vi "Auto Near Switch.vi"(10 "Right?":bool) -> ()   [LabVIEW 2017]
uses:
  Auto switch direita.ctl
  LabVIEW_is_Under_Control.lib/Util/Unpack Gamepad/Button Cluster.ctl
  Team Code/Robot Global Data.vi
panel:
  in  "Delay fwd 2":i32=200
  in  "DistanceAfterTurn":dbl=40.0
  in  "Delay Turn":i32=200
  in  "Turn":dbl=-90.0 format="%#_13g"
  in  "Time to wait (min 50ms)":dbl=50.0
  in  "Delay Fwd":i32=500
  in  "DistanceSwitch":dbl=400.0
  out "auto state":T1=enum."Girando"
  # "AINDA FALTA ADCIONAR:\n\n- Gatilho que troque de estado caso o tempo limite tenha passado\n\n-Algo que detecte um mal funcionamento do navx, e ignore o sinal dele para fazer o auto."
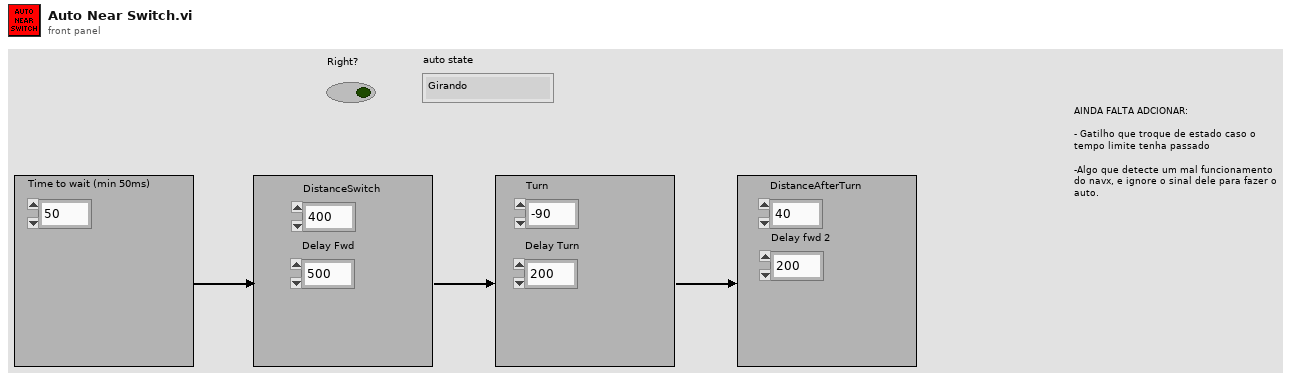
[diagram p1: front panel]
types:
  T1 = typedef "Auto switch direita.ctl" = enum16{"Zerandosensor", "Girando", "Andando", "Jogando", "Andando2", "Finalizando", "Zerandosensor2"}
  T2 = cluster{"proportional gain (Kc)":dbl, "integral time (Ti, min)":dbl, "derivative time (Td, min)":dbl}
  T3 = typedef "Button Cluster.ctl" = cluster{"Buttons[0]":bool, "Buttons[1]":bool, "Buttons[2]":bool, "Buttons[3]":bool, "Buttons[4]":bool, "Buttons[5]":bool, "Buttons[6]":bool, "Buttons[7]":bool, "Buttons[8]":bool, "Buttons[9]":bool}
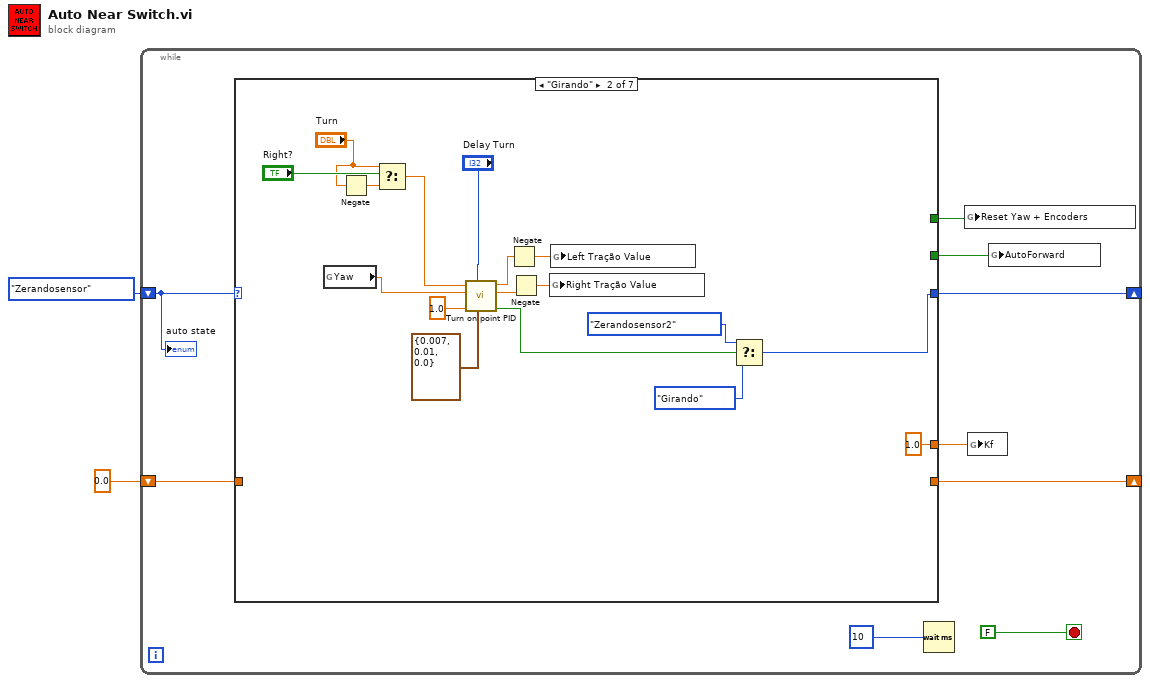
[diagram p0: block diagram]
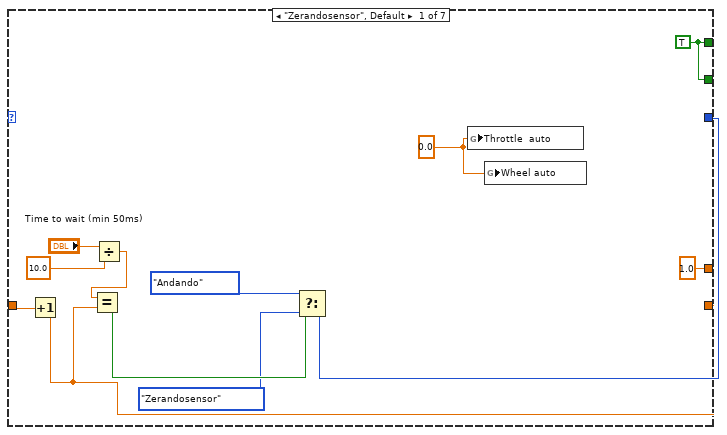
[diagram p2: hidden frame]
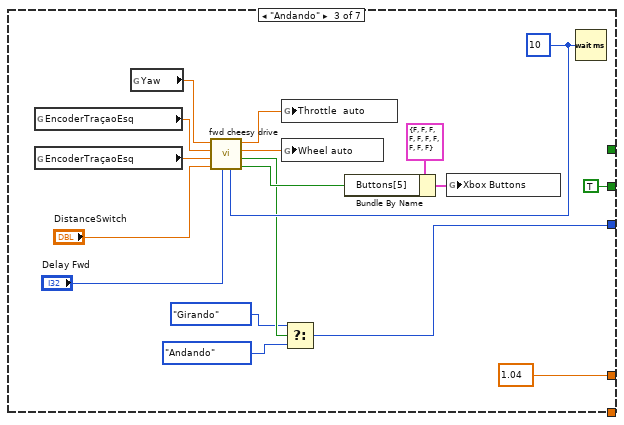
[diagram p3: hidden frame]
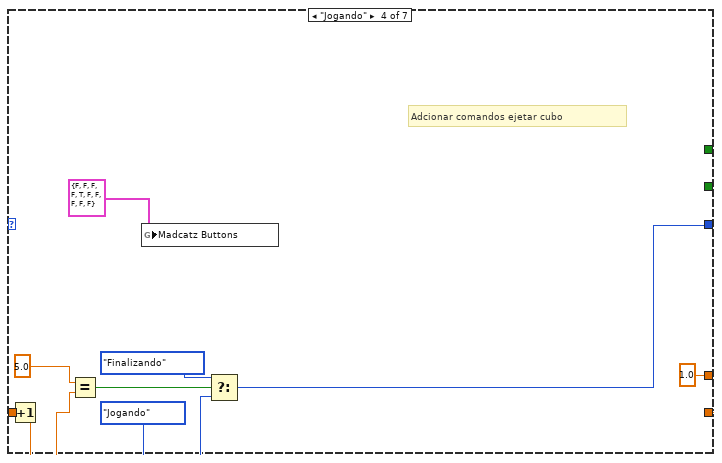
[diagram p4: hidden frame]
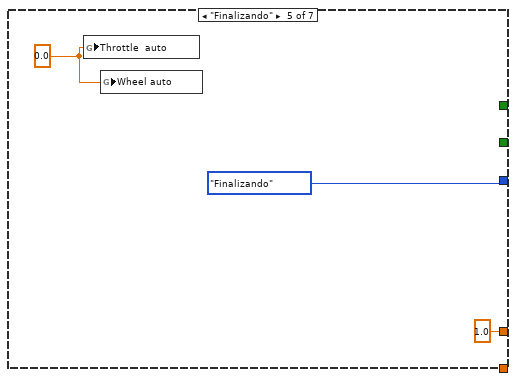
[diagram p5: hidden frame]
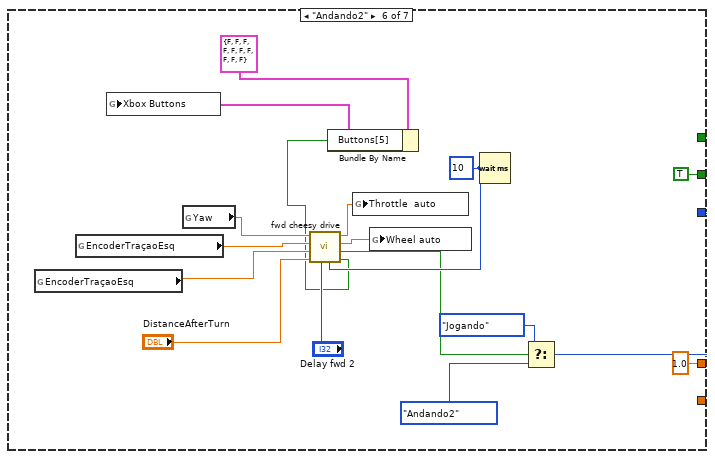
[diagram p6: hidden frame]
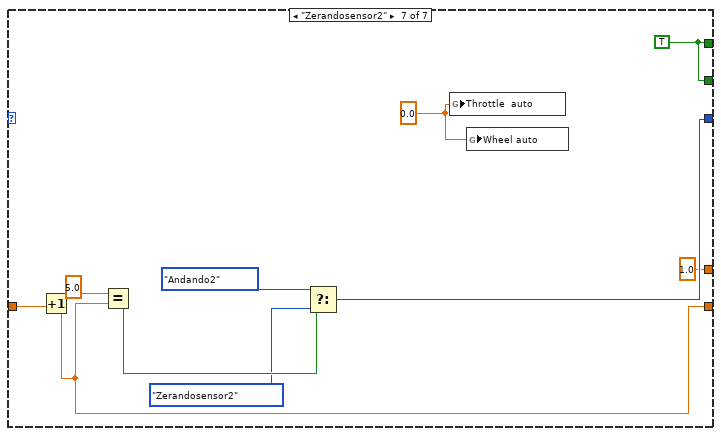
[diagram p7: hidden frame]
diagram:
  n1 = while {
    shift-right: [w7] -> _
    shift-left: Auto_switch_direita."Zerandosensor" -> [w5]
    shift-right: [w8] -> _
    shift-left: 0.0 -> [w9]
    stop <- FALSE stop-if-true
    n2 = case shown="\"Girando\"" w5 {
      tunnel: w9 -> [w23 _ _ w65 _ _ w88]
      tunnel: [w21 _ _ w62 _ _ w89] -> w8
      tunnel: [w20 w38 w45 w61 Auto_switch_direita."Finalizando" w72 w90] -> w7
      tunnel: [w17 _ _ _ _ _ w95] -> w4
      tunnel: [w17 _ TRUE _ _ TRUE w95] -> w6
      tunnel: [1.0 1.0 1.04 1.0 1.0 1.0 1.0] -> w3
      frame "Zerandosensor", Default {
        w16 = 0.0
        w17 = TRUE
        n3 = Increment(x=w23) -> (x+1=w21:dbl)
        n4 = Divide(x="Time to wait (min 50ms)", y=10.0) -> (x/y=w12:dbl)
        n5 = Equal?(x=w12, y=w21) -> (x = y?=w22:bool)
        n6 = Select(t=Auto_switch_direita."Andando", s=w22, f=Auto_switch_direita."Zerandosensor") -> (s? t:f=w20:T1)
        n7 = global write "Robot Global Data.vi" "Throttle  auto"(w16) -> ()
        n8 = global write "Robot Global Data.vi" "Wheel auto"(w16) -> ()
      }
      frame "Girando" {
        n9 = global read "Robot Global Data.vi" "Yaw"() -> (w31:dbl)
        n10 = Negate(x="Turn") -> (-x=w26:dbl)
        n11 = Select(t="Turn", s="Right?", f=w26) -> (s? t:f=w24:dbl)
        n12 = call "Turn on point PID.vi"("Gains"=T2 {"proportional gain (Kc)"=0.007, "integral time (Ti, min)"=0.01, "derivative time (Td, min)"=0.0}, "Time to stop"="Delay Turn", "Precision"=1.0, "Yaw"=w31, "Setpoint(degrees)"=w24) -> ("Finished?"=w39:bool, "PWM right"=w34:dbl, "PWM left"=w35:dbl)  [unwired: 4 in]
        n13 = Negate(x=w35) -> (-x=w30:dbl)
        n14 = Negate(x=w34) -> (-x=w29:dbl)
        n15 = global write "Robot Global Data.vi" "Right Tração Value"(w29) -> ()
        n16 = global write "Robot Global Data.vi" "Left Tração Value"(w30) -> ()
        n17 = Select(t=Auto_switch_direita."Zerandosensor2", s=w39, f=Auto_switch_direita."Girando") -> (s? t:f=w38:T1)
      }
      frame "Andando" {
        w53 = u32 10 ("milliseconds to wait")
        n18 = global read "Robot Global Data.vi" "EncoderTraçaoEsq"() -> (w55:dbl)
        n19 = global read "Robot Global Data.vi" "EncoderTraçaoEsq"() -> (w56:dbl)
        n20 = global read "Robot Global Data.vi" "Yaw"() -> (w57:dbl)
        n21 = call "fwd cheesy drive.vi"("Loop Timer"=w53, "Time to stop"="Delay Fwd", "Distance"="DistanceSwitch", "Encoder Left"=w56, "Encoder Right"=w55, "Yaw"=w57) -> ("Finished distance"=w47:bool, "Both finished"=w46:bool, "Direction"=w51:dbl, "Trottle"=w50:dbl)  [unwired: 2 in]
        n22 = global write "Robot Global Data.vi" "Throttle  auto"(w50) -> ()
        n23 = global write "Robot Global Data.vi" "Wheel auto"(w51) -> ()
        n24 = Select(t=Auto_switch_direita."Girando", s=w46, f=Auto_switch_direita."Andando") -> (s? t:f=w45:T1)
        n25 = Bundle By Name(cluster=T3 {"Buttons[0]"=FALSE, "Buttons[1]"=FALSE, "Buttons[2]"=FALSE, "Buttons[3]"=FALSE, "Buttons[4]"=FALSE, "Buttons[5]"=FALSE, "Buttons[6]"=FALSE, "Buttons[7]"=FALSE, "Buttons[8]"=FALSE, "Buttons[9]"=FALSE} ("Xbox Buttons"), "Buttons[5]"=w47) -> (w48:T3)
        n26 = global write "Robot Global Data.vi" "Xbox Buttons"(w48) -> ()
        n27 = Wait (ms)(milliseconds to wait=w53) -> ()  [unwired: 1 out]
      }
      frame "Jogando" {
        # "Adcionar comandos ejetar cubo"
        n28 = Increment(x=w65) -> (x+1=w62:dbl)
        n29 = Equal?(x=5.0, y=w62) -> (x = y?=w63:bool)
        n30 = global write "Robot Global Data.vi" "Madcatz Buttons"(T3 {"Buttons[0]"=FALSE, "Buttons[1]"=FALSE, "Buttons[2]"=FALSE, "Buttons[3]"=FALSE, "Buttons[4]"=TRUE, "Buttons[5]"=FALSE, "Buttons[6]"=FALSE, "Buttons[7]"=FALSE, "Buttons[8]"=FALSE, "Buttons[9]"=FALSE} ("Madcatz Buttons")) -> ()
        n31 = Select(t=Auto_switch_direita."Finalizando", s=w63, f=Auto_switch_direita."Jogando") -> (s? t:f=w61:T1)
      }
      frame "Finalizando" {
        w67 = 0.0
        n32 = global write "Robot Global Data.vi" "Throttle  auto"(w67) -> ()
        n33 = global write "Robot Global Data.vi" "Wheel auto"(w67) -> ()
      }
      frame "Andando2" {
        w82 = u32 10 ("milliseconds to wait")
        n34 = global read "Robot Global Data.vi" "EncoderTraçaoEsq"() -> (w85:dbl)
        n35 = global read "Robot Global Data.vi" "EncoderTraçaoEsq"() -> (w84:dbl)
        n36 = global read "Robot Global Data.vi" "Yaw"() -> (w86:dbl)
        n37 = call "fwd cheesy drive.vi"("Loop Timer"=w82, "Time to stop"="Delay fwd 2", "Distance"="DistanceAfterTurn", "Encoder Left"=w85, "Encoder Right"=w84, "Yaw"=w86) -> ("Finished distance"=w76:bool, "Both finished"=w75:bool, "Direction"=w80:dbl, "Trottle"=w79:dbl)  [unwired: 2 in]
        n38 = Bundle By Name(cluster=T3 {"Buttons[0]"=FALSE, "Buttons[1]"=FALSE, "Buttons[2]"=FALSE, "Buttons[3]"=FALSE, "Buttons[4]"=FALSE, "Buttons[5]"=FALSE, "Buttons[6]"=FALSE, "Buttons[7]"=FALSE, "Buttons[8]"=FALSE, "Buttons[9]"=FALSE} ("Xbox Buttons"), "Buttons[5]"=w76) -> (w77:T3)
        n39 = global write "Robot Global Data.vi" "Xbox Buttons"(w77) -> ()
        n40 = global write "Robot Global Data.vi" "Throttle  auto"(w79) -> ()
        n41 = global write "Robot Global Data.vi" "Wheel auto"(w80) -> ()
        n42 = Wait (ms)(milliseconds to wait=w82) -> ()  [unwired: 1 out]
        n43 = Select(t=Auto_switch_direita."Jogando", s=w75, f=Auto_switch_direita."Andando2") -> (s? t:f=w72:T1)
      }
      frame "Zerandosensor2" {
        w95 = TRUE
        w96 = 0.0
        n44 = Increment(x=w88) -> (x+1=w89:dbl)
        n45 = Equal?(x=5.0, y=w89) -> (x = y?=w93:bool)
        n46 = Select(t=Auto_switch_direita."Andando2", s=w93, f=Auto_switch_direita."Zerandosensor2") -> (s? t:f=w90:T1)
        n47 = global write "Robot Global Data.vi" "Throttle  auto"(w96) -> ()
        n48 = global write "Robot Global Data.vi" "Wheel auto"(w96) -> ()
      }
    }
    n49 = Wait (ms)(milliseconds to wait=u32 10) -> ()  [unwired: 1 out]
    n50 = global write "Robot Global Data.vi" "Reset Yaw + Encoders"(w4) -> ()
    n51 = global write "Robot Global Data.vi" "Kf"(w3) -> ()
    n52 = global write "Robot Global Data.vi" "AutoForward"(w6) -> ()
    "auto state" <- w5
  }
